vi "AutoProceed.vi"() -> ()   [LabVIEW 2016]
panel:
  out "Flip":bool
  out "Auto Proceed":bool
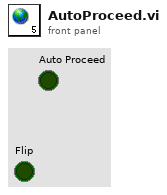
[diagram p1: front panel]
diagram:
